vi "updateTuplaEnDB.vi"(8 "error in":errorcluster, 9 "RawIndexToModify":i32[](array[numeric]), 10 "ItemNames":string[][](array[string]), 11 "claseDB in":refnum<class "claseDB.lvclass">) -> (0 "error out":errorcluster, 3 "claseDB out":refnum<class "claseDB.lvclass">)   [LabVIEW 2014, in "claseDB.lvclass"]
uses:
  claseDB.lvclass
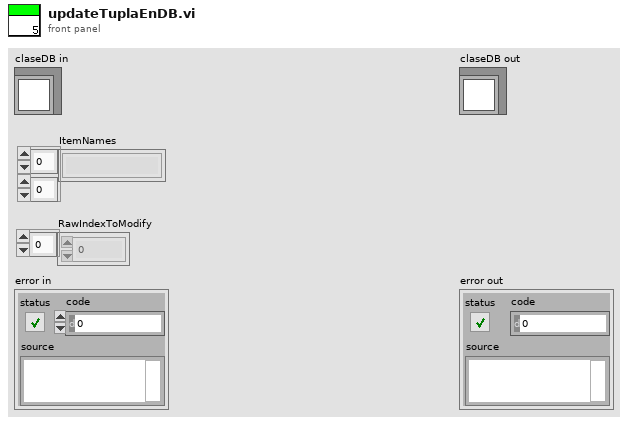
[diagram p1: front panel]
types:
  T1 = cluster{"objetoProduct":cluster{"idProduct":dbl, "od":string, "steelGrade":string, "lote":string, "dateCreate":timestamp, "idRecipe":dbl}, "objetoImage":cluster{"idImage":dbl, "camposDeMedicion":string, "dateCreate":timestamp}, "objetoRecipe":cluster{"idRecipe":dbl, "od":string, "steelGrade":string, "camposDeMedicion":string, "dateCreate":timestamp, "idStadistic":string}, "objetoStadistic":cluster{"idStadistic":dbl, "camposDeMedicion":string, "dateCreate":timestamp}, "objetoMetalRod":cluster{"idRod":dbl, "camposDeMedicion":string, "dateCreate":timestamp, "idProduct":dbl, "idImage":dbl}, "tableToUse":cluster{"useTableProduct":bool, "useTableImage":bool, "useTableRecipe":bool, "useTableStadistic":bool, "useTableMetalRod":bool}}
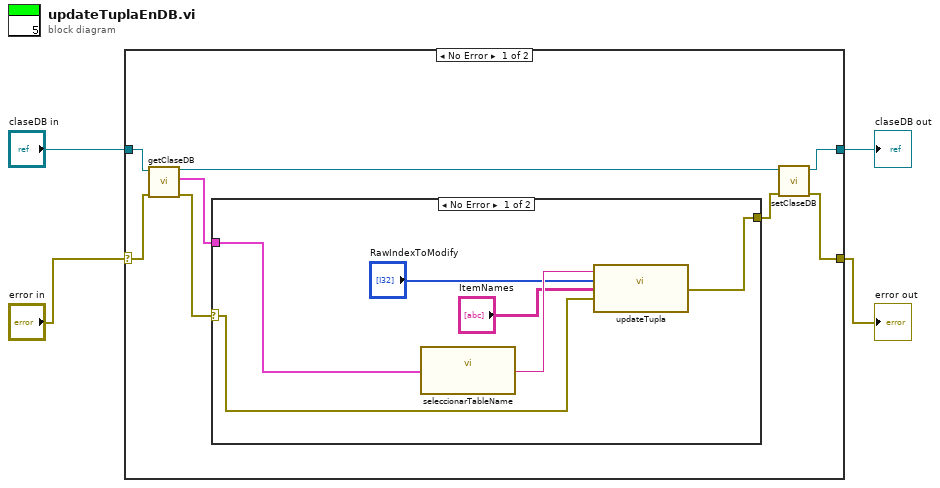
[diagram p0: block diagram]
diagram:
  n1 = case shown="No Error" "error in" {
    selector: "error in" -> [w11 w21]
    tunnel: [w8 w21] -> w3
    tunnel: "claseDB in" -> [w12 w20]
    tunnel: [w9 w20] -> w1
    frame No Error {
      n2 = call "getClaseDB.vi"("error in"=w11, "claseDB.lvclass"=w12) -> ("error out"=w5:errorcluster, "datosClaseDB"=w6:T1, "claseDB.lvclass 2"=w10:refnum<class "claseDB.lvclass">)  [unwired: 7 in]
      n3 = case shown="No Error" w5 {
        selector: w5 -> [w13 w19]
        tunnel: [w17 w19] -> w7
        tunnel: w6 -> [w14 _]
        frame No Error {
          n4 = call "seleccionarTableName.vi"("datosClaseDB in"=w14) -> ("tableNameOut"=w18:string)  [unwired: 10 in]
          n5 = call "updateTupla.vi"("error in"=w13, "ItemNames"="ItemNames", "RawIndexToModify"="RawIndexToModify", "tableName"=w18) -> ("error out"=w17:errorcluster)  [unwired: 7 in]
        }
        frame Error {
        }
      }
      n6 = call "setClaseDB.vi"("error in"=w7, "claseDB in"=w10) -> ("error out"=w8:errorcluster, "claseDB out"=w9:refnum<class "claseDB.lvclass">)  [unwired: 8 in]
    }
    frame Error {
    }
  }
  "claseDB out" <- w1
  "error out" <- w3
